vi "Modbus Write SGL.vi"(7 "Slave Address":u8, 8 "error in (no error)":errorcluster, 9 "Input data float32":sgl, 10 "Register Start Address":u16 format="%x", 11 "VISA resource in":refnum<visa-resource-name>) -> (0 "error out":errorcluster, 3 "VISA resource out":refnum<visa-resource-name>)   [LabVIEW 2023, in "Voegtlin_NI_SMART_Modbus_Drivers.lvlib"]
doc: "Schreibe einen float32-Wert an die angegebene Startadresse des selektierten Geraetes.\nDer COM-Port muss dazu initialisiert sein (benutze\" Modbus Init.vi\")."
uses:
  Voegtlin_NI_SMART_Modbus_Drivers.lvlib
  Enums/Modbus Comm.ctl
panel:
  out "U16 input data to write\n(array)":u16[](array[numeric])
  # "Input Data"
  # "Internal Data"
  # "Output Data"
  # "(Inputmaske in HEX)"
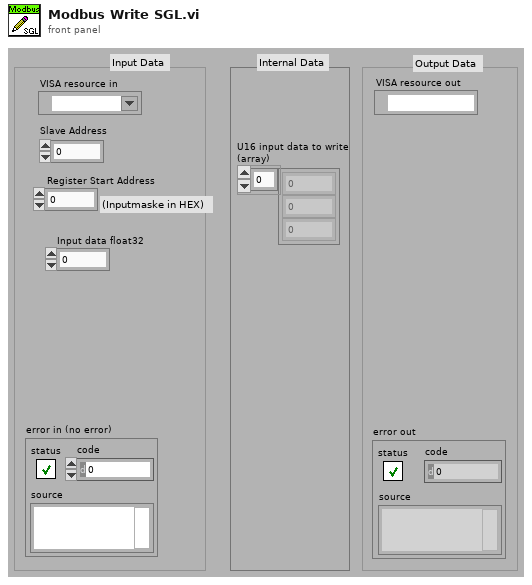
[diagram p1: front panel]
types:
  T1 = typedef "Voegtlin_NI_SMART_Modbus_Drivers.lvlib/Modbus Comm.ctl" = enum16{"Init", "Read", "Write", "Exit"}
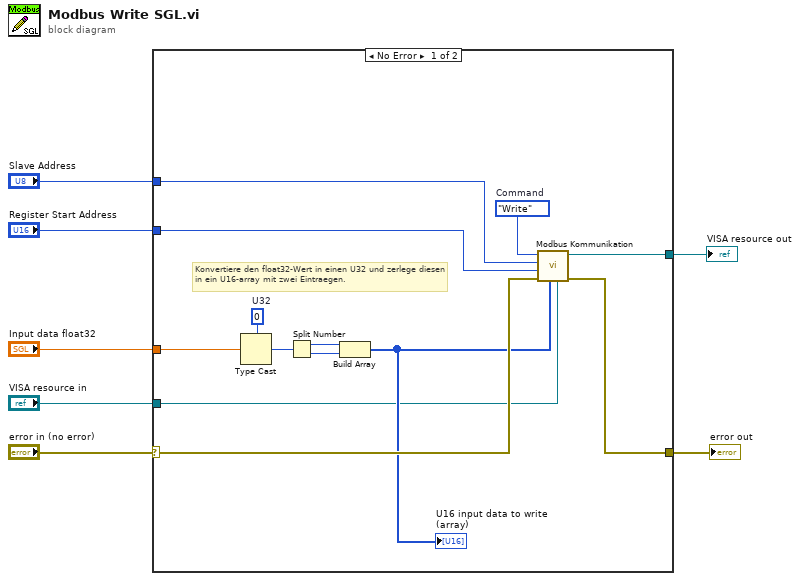
[diagram p0: block diagram]
diagram:
  n1 = case shown="No Error" "error in (no error)" {
    selector: "error in (no error)" -> [w13 w22]
    tunnel: [w19 w22] -> w7
    tunnel: "Register Start Address" -> [w11 _]
    tunnel: "Input data float32" -> [w14 _]
    tunnel: "Slave Address" -> [w10 _]
    tunnel: "VISA resource in" -> [w9 w21]
    tunnel: [w8 w21] -> w1
    frame No Error {
      w18 = u32 0  # U32
      w20 = Modbus_Comm."Write"  # Command
      # "Konvertiere den float32-Wert in einen U32 und zerlege diesen in ein U16-array mit zwei Eintraegen."
      n2 = Type Cast(type=w18, x=w14) -> (*(type *) &x=w17:u32)
      n3 = Split Number(x=w17) -> (hi(x)=w16:u16, lo(x)=w15:u16)
      n4 = Build Array(w16, w15) -> (w12:u16[])
      "U16 input data to write\n(array)" <- w12
      n5 = call "Modbus Kommunikation.vi"("VISA resource in"=w9, "Data In / #Reads [U16]"=w12, "error in (no error)"=w13, "Register Start Address"=w11, "Slave Address"=w10, "Command"=w20) -> ("error out"=w19:errorcluster, "VISA resource out"=w8:refnum<visa-resource-name>)  [unwired: 3 in, 1 out]
    }
    frame Error {
    }
  }
  "error out" <- w7
  "VISA resource out" <- w1
